vi "_Read ADC.vi"(1 "Channel #":u8) -> ()   [LabVIEW 2012]
uses:
  Type/_FPGA Chip Type.ctl
  <vilib>/rvi/eio/common/nirviEmuTemplateMethod_errors.vi
  <vilib>/rvi/DataTransferAndStorage/Container/Common/niFpgaContainerGetUniqueNameForEmu.vi
  <vilib>/rvi/Memory/Memory_Emulation/niFpgaMemoryEmulationCacheClearOnFirstRun.vi
  <vilib>/rvi/Memory/Memory_Emulation/nirvimemoryEmulationManagerCache_MakeExclusive.vi
  <vilib>/rvi/Memory/Memory_Emulation/niFpgaMemoryEmulationValidateCache.vi
  <vilib>/rvi/Memory/Memory_Emulation/nirvimemoryEmulationManagerCache_ReleaseExclusive.vi
  <vilib>/rvi/Memory/Memory_Emulation/nirvimemoryEmulationManagerCache_InsertValue.vi
  <vilib>/Utility/error.llb/Clear Errors.vi
  <vilib>/rvi/Emulation/niFpgaSctlEmulationGetInTimedLoop.vi
  <vilib>/rvi/Memory/Memory_Emulation/nirvimemoryEmulationManagerCache_GetValue.vi
  <vilib>/rvi/Memory/Memory_Emulation/nirvimemoryEmulationManagerCache_SetValue.vi
  <vilib>/rvi/Emulation/niFpgaSctlEmulationResourceMgr.vi
  <vilib>/eio/EIONode/EIONode.xnode
  <vilib>/rvi/DataTransferAndStorage/Container/XNode/niFpgaContainer.xnode
  <vilib>/rvi/Memory/Memory_Emulation/nirvimemoryEmulation.vi
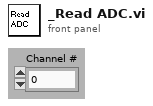
[diagram p1: front panel]
types:
  T1 = typedef "_FPGA Chip Type.ctl" = enum8{"None", "ADC1", "ADC2", "ADC3", "ADC4", "ADC5", "ADC6", "ADC7", "ADC8", "ADC9", "ADC10", "ADC11", "ADC12", "ADC13", "DAC1", "DAC2", "DAC3", "DAC4", "DAC5", "LENS1", "LENS2", "LENS3", "LENS4", "LENS5", "LENS6", "LENS7", "MASS1", "MASS2", "MASS3", "MASS4", "MASS5", "OSC1", "OSC2", "OSC3", "LATCH1", "LATCH2", "LATCH3", "LATCH4", "PIC1", "PIC2", "PIC3", "PIC4"}
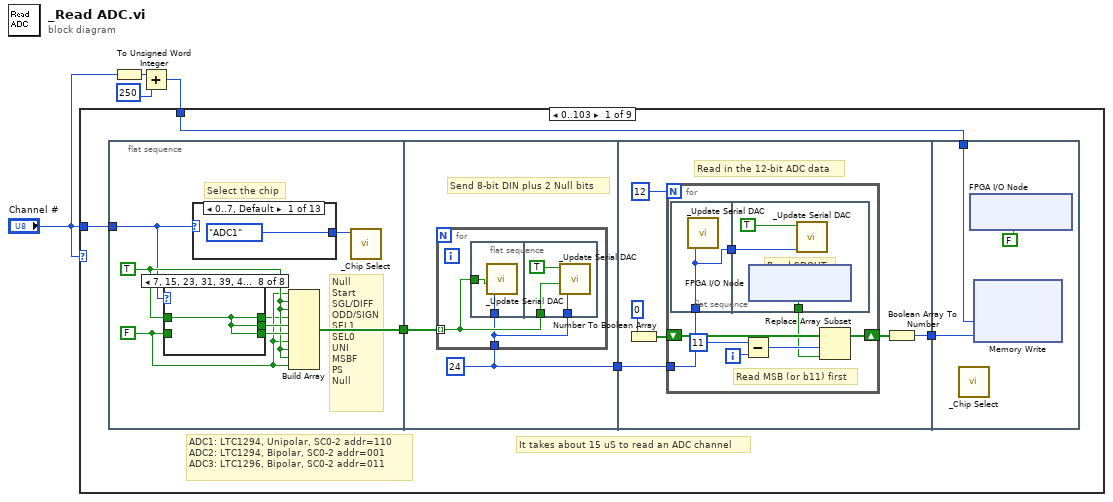
[diagram p0: block diagram]
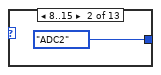
[diagram p9: hidden frame]
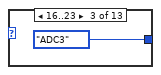
[diagram p10: hidden frame]
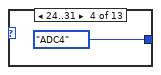
[diagram p11: hidden frame]
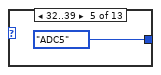
[diagram p12: hidden frame]
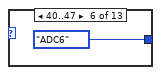
[diagram p13: hidden frame]
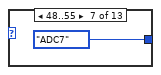
[diagram p14: hidden frame]
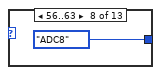
[diagram p15: hidden frame]
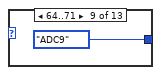
[diagram p16: hidden frame]
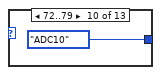
[diagram p17: hidden frame]
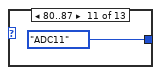
[diagram p18: hidden frame]
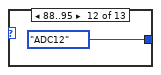
[diagram p19: hidden frame]
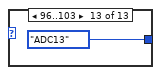
[diagram p20: hidden frame]
diagram:
  n1 = To Unsigned Word Integer(number="Channel #") -> (unsigned 16bit integer=w4:u16)
  n2 = Add(x=w4, y=u16 250 ("Timeout (-1 for no timeout)")) -> (x+y=w2:u16)
  n3 = case shown="0..103" "Channel #" {
    tunnel: "Channel #" -> [w7 w80 w83 _ _ _ _ _ _]
    tunnel: w2 -> [w6 w79 _ _ w93 w96 w99 w102 w105]
    frame 0..103 {
      # "It takes about 15 uS to read an ADC channel"
      # "ADC1: LTC1294, Unipolar, SC0-2 addr=110\nADC2: LTC1294, Bipolar, SC0-2 addr=001\nADC3: LTC1296, Bipolar, SC0-2 addr=011"
      n4 = flat-sequence {
        tunnel: [w15] -> w9
        tunnel: w7 -> [w10]
        tunnel: w9 -> [w46]
        tunnel: [w45] -> w5
        tunnel: [w55] -> w8
        tunnel: w5 -> [w54]
        tunnel: w8 -> [w74]
        tunnel: w6 -> [w73]
        frame #0 {
          w12 = FALSE
          w14 = TRUE
          # "Null\nStart\nSGL/DIFF\nODD/SIGN\nSEL1\nSEL0\nUNI\nMSBF\nPS\nNull"
          # "Select the chip"
          n5 = case shown="7, 15, 23, 31, 39, 47, 55, 63, 71, 79, 87, 95, 103" w10 {
            tunnel: [w18 w20 w22 w24 w25 w28 w29 w31] -> w11
            tunnel: [w18 w19 w22 w23 w26 w28 w30 w31] -> w17
            tunnel: [w18 w19 w21 w24 w25 w27 w30 w31] -> w16
            tunnel: w14 -> [_ w20 w21 w24 w26 w28 w30 w31]
            tunnel: w12 -> [w18 w19 w22 w23 w25 w27 w29 _]
            frame 0, 8, 16, 24, 32, 40, 48, 56, 64, 72, 80, 88, 96, Default {
            }
            frame 1, 9, 17, 25, 33, 41, 49, 57, 65, 73, 81, 89, 97 {
            }
            frame 2, 10, 18, 26, 34, 42, 50, 58, 66, 74, 82, 90, 98 {
            }
            frame 3, 11, 19, 27, 35, 43, 51, 59, 67, 75, 83, 91, 99 {
            }
            frame 4, 12, 20, 28, 36, 44, 52, 60, 68, 76, 84, 92, 100 {
            }
            frame 5, 13, 21, 29, 37, 45, 53, 61, 69, 77, 85, 93, 101 {
            }
            frame 6, 14, 22, 30, 38, 46, 54, 62, 70, 78, 86, 94, 102 {
            }
            frame 7, 15, 23, 31, 39, 47, 55, 63, 71, 79, 87, 95, 103 {
            }
          }
          n6 = case shown="0..7, Default" w10 {
            tunnel: [_FPGA_Chip_Type."ADC1" ("ChipType") _FPGA_Chip_Type."ADC2" ("ChipType") _FPGA_Chip_Type."ADC3" ("ChipType") _FPGA_Chip_Type."ADC4" ("ChipType") _FPGA_Chip_Type."ADC5" ("ChipType") _FPGA_Chip_Type."ADC6" ("ChipType") _FPGA_Chip_Type."ADC7" ("ChipType") _FPGA_Chip_Type."ADC8" ("ChipType") _FPGA_Chip_Type."ADC9" ("ChipType") _FPGA_Chip_Type."ADC10" ("ChipType") _FPGA_Chip_Type."ADC11" ("ChipType") _FPGA_Chip_Type."ADC12" ("ChipType") _FPGA_Chip_Type."ADC13" ("ChipType")] -> w13
            frame 0..7, Default {
            }
            frame 8..15 {
            }
            frame 16..23 {
            }
            frame 24..31 {
            }
            frame 32..39 {
            }
            frame 40..47 {
            }
            frame 48..55 {
            }
            frame 56..63 {
            }
            frame 64..71 {
            }
            frame 72..79 {
            }
            frame 80..87 {
            }
            frame 88..95 {
            }
            frame 96..103 {
            }
          }
          n7 = Build Array(w12, w14, w14, w11, w17, w16, w12, w14, w14, w12) -> (w15:bool[])
          n8 = call "_Chip Select.vi"("ChipType"=w13) -> ()  [unwired: 1 in, 6 out]
        }
        frame #1 {
          w45 = u8 24 ("Wait(12Ticks)")
          # "Send 8-bit DIN plus 2 Null bits"
          n9 = for {
            tunnel: w46 -> [w48] mode=indexing
            tunnel: w45 -> [w47]
            n10 = flat-sequence {
              tunnel: w48 -> [w50]
              tunnel: w47 -> [w49]
              tunnel: w48 -> [w53]
              tunnel: w47 -> [w51]
              frame #0 {
                n11 = call "_Update Serial DAC.vi"("Wait(12Ticks)"=w49, "DIN (F)"=w50) -> ()  [unwired: 2 in, 4 out]
              }
              frame #1 {
                n12 = call "_Update Serial DAC.vi"("Wait(12Ticks)"=w51, "DIN (F)"=w53, "Clock (F)"=TRUE ("Clock")) -> ()  [unwired: 1 in, 4 out]
              }
            }
          }
        }
        frame #2 {
          # "Read in the 12-bit ADC data"
          n13 = Number To Boolean Array(number=u16 0) -> (Boolean array=w57:bool[])
          n14 = for {
            N: 12 -> [_]
            shift-right: [w66] -> w56
            shift-left: w57 -> [w67]
            tunnel: w54 -> [w61]
            i -> [w65]
            # "Read MSB (or b11) first"
            n15 = flat-sequence {
              tunnel: w61 -> [w68]
              tunnel: [w68] -> w60
              tunnel: [w70] -> w62
              tunnel: w60 -> [w69]
              frame #0 {
                n16 = call "_Update Serial DAC.vi"("Wait(12Ticks)"=w68) -> ()  [unwired: 3 in, 4 out]
              }
              frame #1 {
                # "Read SDOUT"
                n17 = xnode "FPGA I/O Node"() -> ("Port0/DIO7"=w70:bool)  [unwired: 1 in, 1 out]
                n18 = call "_Update Serial DAC.vi"("Wait(12Ticks)"=w69, "Clock (F)"=TRUE ("Clock")) -> ()  [unwired: 2 in, 4 out]
              }
            }
            n19 = Subtract(x=11, y=w65) -> (x-y=w63:i32)
            n20 = Replace Array Subset(array=w67, new element=w62, index=w63) -> (w66:bool[])
          }
          n21 = Boolean Array To Number(Boolean array=w56) -> (number=w55:u16)
        }
        frame #3 {
          n22 = call "_Chip Select.vi"() -> ()  [unwired: 2 in, 6 out]
          n23 = xnode "FPGA I/O Node"("Port1/DIO0"=FALSE) -> ()  [unwired: 1 in, 1 out]
          n24 = xnode ("Memory Write")("Address"=w73, "Data"=w74) -> ()  [unwired: 1 in, 1 out]
        }
      }
    }
    frame 104..110 {
      # "Read PIC channels"
      n25 = xnode ("Memory Read")("Address"=w79) -> ("Data"=w76:u32)  [unwired: 1 in, 1 out]
      n26 = Split Number(x=w76) -> (hi(x)=w75:u16)  [unwired: 1 out]
      n27 = Subtract(x=w80, y=u8 24) -> (x-y=w77:u8)
      n28 = call "_Set 1 DAC Value.vi"("DAC"=w75, "Ch#"=w77) -> ()  [unwired: 2 out]
    }
    frame 113, 114 {
      # "Read Source ID"
      n29 = Subtract(x=w83, y=u8 24) -> (x-y=w81:u8)
      n30 = while {
        tunnel: w81 -> [w91]
        i -> [w85]
        stop <- w88 stop-if-true
        w84 = u8 2 ("upper limit")
        n31 = call "_Set 1 DAC Value.vi"("Ch#"=w91) -> ("PIC Monitor"=w90:u8)  [unwired: 1 in, 1 out]
        n32 = Greater Or Equal?(x=w85, y=w84) -> (x >= y?=w86:bool)
        n33 = In Range and Coerce(upper limit=w84, x=w90, lower limit=u8 0) -> (In Range?=w87:bool)  [unwired: 1 out]
        n34 = Or(x=w87, y=w86) -> (x .or. y?=w88:bool)
      }
    }
    frame 115, Default {
      # "No need to read the -ve PIC channels\nas they are the same as the +ve channels"
    }
    frame 119 {
      # "Read VAC Gauge"
      n35 = call "_Read VAC Gauge.vi"() -> ("DAC"=w92:u8)
      n36 = xnode ("Memory Write")("Address"=w93, "Data"=w92) -> ()  [unwired: 1 in, 1 out]
    }
    frame 120 {
      # "Read Card Cage Door Interlock"
      n37 = xnode "FPGA I/O Node"() -> ("Port6/DIO7"=w95:bool)  [unwired: 1 in, 1 out]
      n38 = Boolean To (0,1)(Boolean=w95) -> (0, 1=w94:i16)
      n39 = xnode ("Memory Write")("Address"=w96, "Data"=w94) -> ()  [unwired: 1 in, 1 out]
    }
    frame 121 {
      # "Read Vacuum Ready"
      n40 = xnode "FPGA I/O Node"() -> ("Port0/DIO6"=w98:bool)  [unwired: 1 in, 1 out]
      n41 = Boolean To (0,1)(Boolean=w98) -> (0, 1=w97:i16)
      n42 = xnode ("Memory Write")("Address"=w99, "Data"=w97) -> ()  [unwired: 1 in, 1 out]
    }
    frame 126 {
      # "LC1 In"
      n43 = xnode "FPGA I/O Node"() -> ("Port5/DIO7"=w101:bool)  [unwired: 1 in, 1 out]
      n44 = Boolean To (0,1)(Boolean=w101) -> (0, 1=w100:i16)
      n45 = xnode ("Memory Write")("Address"=w102, "Data"=w100) -> ()  [unwired: 1 in, 1 out]
    }
    frame 127 {
      # "LC2 In"
      n46 = xnode "FPGA I/O Node"() -> ("Port6/DIO0"=w104:bool)  [unwired: 1 in, 1 out]
      n47 = Boolean To (0,1)(Boolean=w104) -> (0, 1=w103:i16)
      n48 = xnode ("Memory Write")("Address"=w105, "Data"=w103) -> ()  [unwired: 1 in, 1 out]
    }
  }
